vi "Overlay Game Object.vi"(7 "Color":u32, 8 "error in (no error)":errorcluster, 9 "Name":string, 10 "Object":T1, 11 "Image In":T2) -> (0 "error out":errorcluster, 3 "Image Out":T2)   [LabVIEW 2018]
uses:
  <vilib>/vision/Image Controls.llb/IMAQ Image.ctl
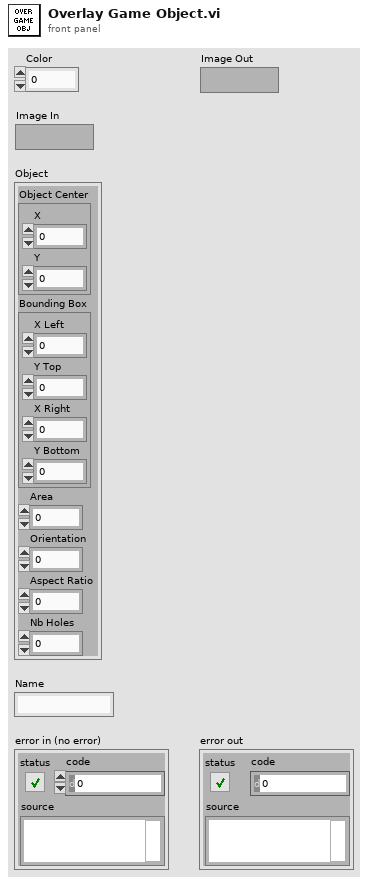
[diagram p1: front panel]
types:
  T1 = cluster{"Object Center":cluster{"X":sgl, "Y":sgl}, "Bounding Box":cluster{"X Left":i32, "Y Top":i32, "X Right":i32, "Y Bottom":i32}, "Area":sgl, "Orientation":sgl, "Aspect Ratio":sgl, "Nb Holes":i32}
  T2 = typedef "IMAQ Image.ctl" = refnum<image>
  T3 = cluster{"X Left":i32, "Y Top":i32, "X Right":i32, "Y Bottom":i32}
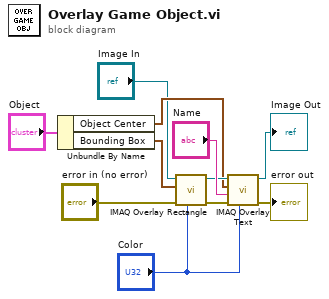
[diagram p0: block diagram]
diagram:
  n1 = Unbundle By Name("Object") -> ("Object Center"=w5:cluster{"X":sgl, "Y":sgl}, "Bounding Box"=w2:T3)
  n2 = call "IMAQ Overlay Rectangle"("Color"="Color", "error in (no error)"="error in (no error)", "Rectangle"=w2, "Image"="Image In") -> ("error out"=w6:errorcluster, "Image Out"=w7:T2)  [unwired: 6 in]
  n3 = call "IMAQ Overlay Text"("Text Color (black)"="Color", "error in (no error)"=w6, "String"="Name", "Origin"=w5, "Image"=w7) -> ("error out"=→"error out":errorcluster, "Image Out"=→"Image Out":T2)  [unwired: 5 in]
